vi "Kinetic Law Processor.vi"(5 "Kinetic Law":string, 11 "error in (no error)":errorcluster) -> (4 "No. of Operators":i32, 6 "No. of Operands":i32, 8 "Parsed array":string[](array[string]), 10 "Tagged String":string, 15 "error out":errorcluster)   [LabVIEW 2014]
doc: "This VI takes \"kinetic Law\" (enclosed in <apply>, </apply> tags) as input and parse it with unique tags. Currently, following five math functions are supported:\n+, - , /, *, pow\n\nDesigned by HB\nhaba@dtu.dk"
panel:
  out "result":i32
  out "flag":i32
  out "Temp_Strng":string
  out "App_Cnt":i32
  # "SOP3 pow SOP4 * SOP5 / kr_f kr_r EOP5 LacI EOP4 nc EOP3"
  # "pow ( (kr_f/kr_r)*LacI, nc)"
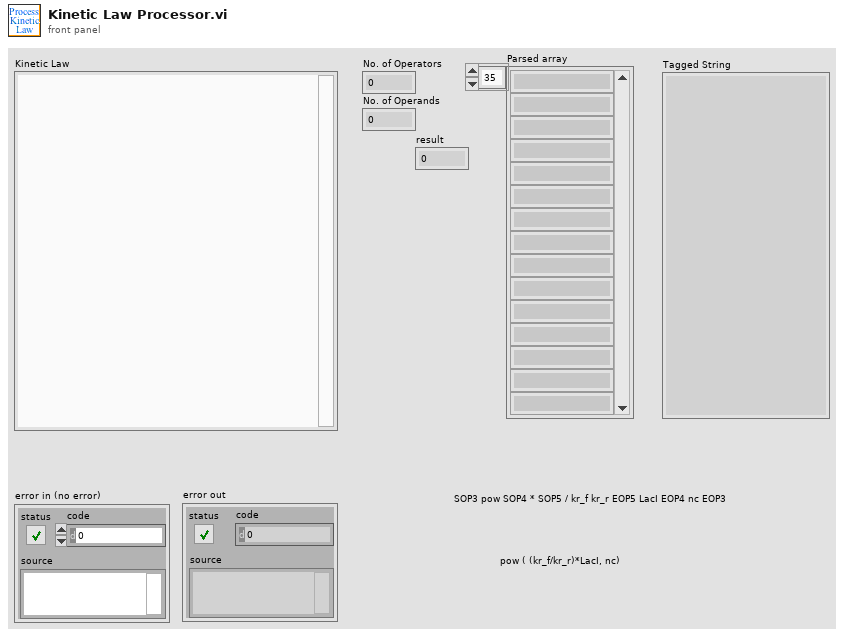
[diagram p1: front panel]
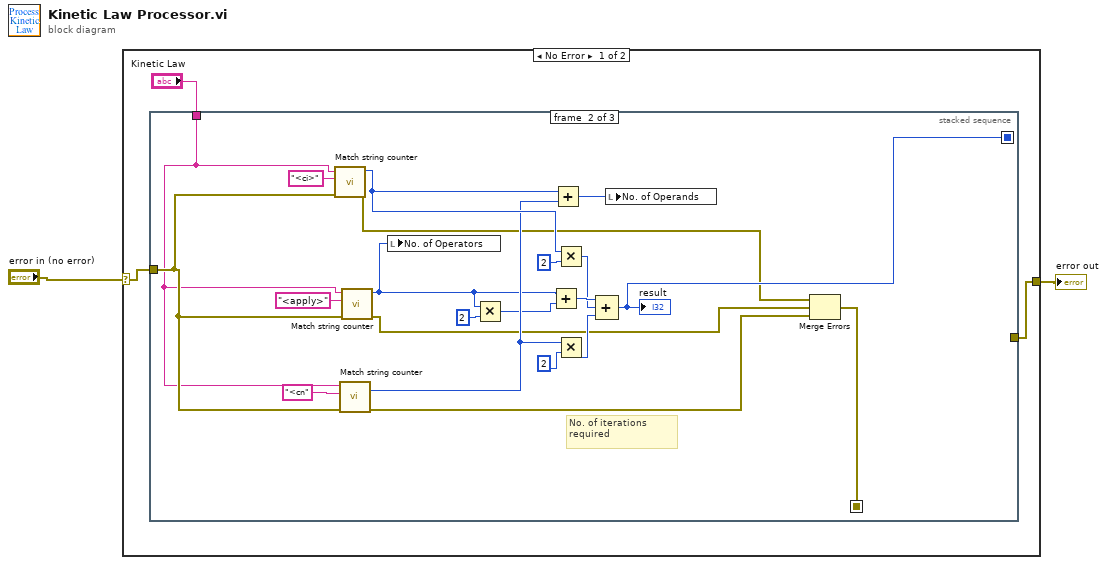
[diagram p0: block diagram]
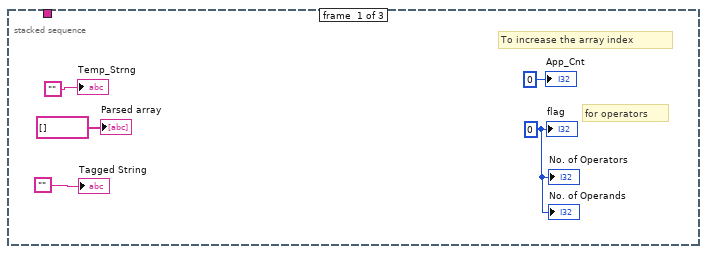
[diagram p2: hidden frame]
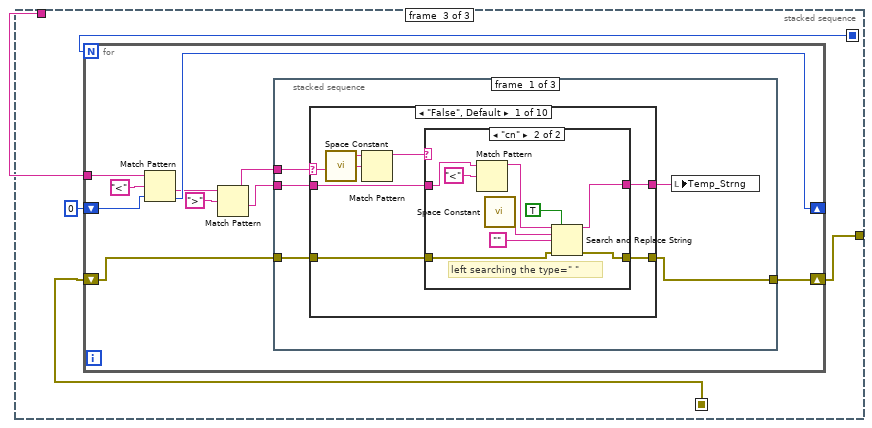
[diagram p3: hidden frame]
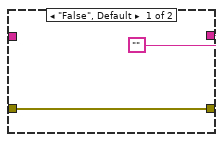
[diagram p4: hidden frame]
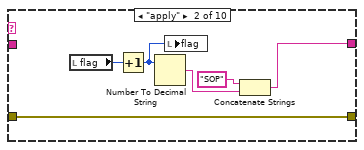
[diagram p5: hidden frame]
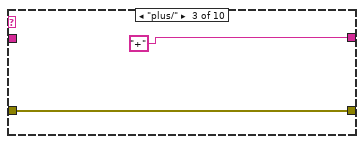
[diagram p6: hidden frame]
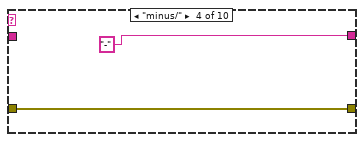
[diagram p7: hidden frame]
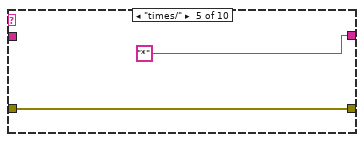
[diagram p8: hidden frame]
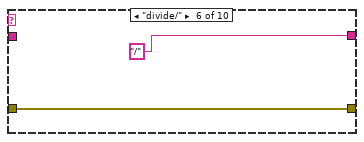
[diagram p9: hidden frame]
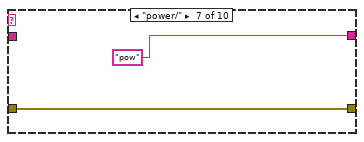
[diagram p10: hidden frame]
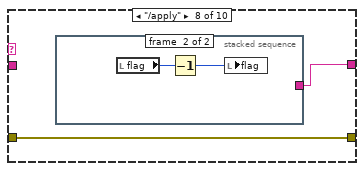
[diagram p11: hidden frame]
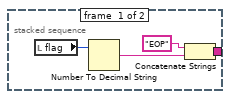
[diagram p12: hidden frame]
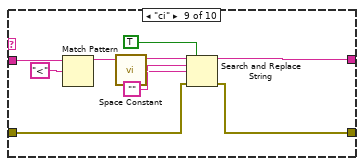
[diagram p13: hidden frame]
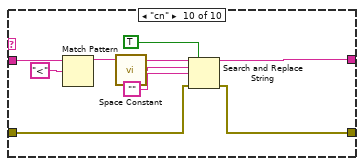
[diagram p14: hidden frame]
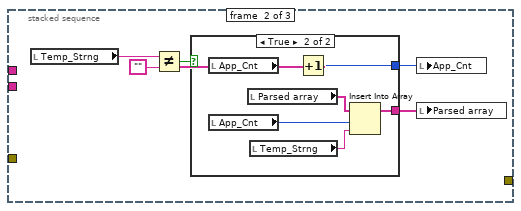
[diagram p15: hidden frame]
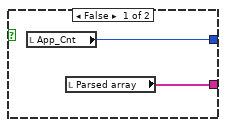
[diagram p16: hidden frame]
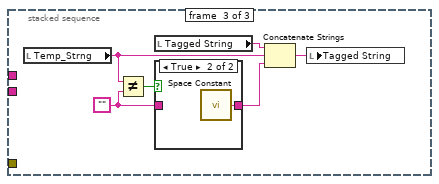
[diagram p17: hidden frame]
diagram:
  n1 = case shown="No Error" "error in (no error)" {
    selector: "error in (no error)" -> [w3 w133]
    tunnel: [w4 w133] -> w2
    frame No Error {
      n2 = stacked-sequence {
        seq-local: [_ w23 _] -> [_ _ w34]
        seq-local: [_ w12 _] -> [_ _ w33]
        tunnel: "Kinetic Law" -> [_ w11 w35]
        tunnel: w3 -> [_ w16 _]
        tunnel: [_ _ w32] -> w4
        frame #0 {
          w6 = 0 ("App_Cnt")
          # "To increase the array index"
          # "for operators"
          "App_Cnt" <- 0 ("App_Cnt")
          "Parsed array" <- string[] []
          "flag" <- w6
          "Temp_Strng" <- ""
          "Tagged String" <- ""
          "No. of Operators" <- w6
          "No. of Operands" <- w6
        }
        frame #1 {
          # "No. of iterations \nrequired"
          n3 = call "Match string counter.vi"("error in (no error)"=w16, "Match String"="<ci>", "Input string"=w11) -> ("error out"=w15:errorcluster, "Count"=w25:i32)  [unwired: 7 in]
          n4 = call "Match string counter.vi"("error in (no error)"=w16, "Match String"="<cn", "Input string"=w11) -> ("error out"=w13:errorcluster, "Count"=w24:i32)  [unwired: 7 in]
          n5 = call "Match string counter.vi"("error in (no error)"=w16, "Match String"="<apply>", "Input string"=w11) -> ("error out"=w14:errorcluster, "Count"=w17:i32)  [unwired: 7 in]
          n6 = local write "No. of Operators"(w17) -> ()
          n7 = Multiply(x=w17, y=2) -> (x*y=w18:i32)
          n8 = Add(x=w17, y=w18) -> (x+y=w30:i32)
          n9 = Add(x=w25, y=w24) -> (x+y=w22:i32)
          n10 = Multiply(x=w25, y=2) -> (x*y=w28:i32)
          n11 = Multiply(x=w24, y=2) -> (x*y=w26:i32)
          n12 = Compound Arithmetic op=ADD(w30, w28, w26) -> (w23:i32)
          "result" <- w23
          n13 = local write "No. of Operands"(w22) -> ()
          n14 = Merge Errors(w15, w14, w13) -> (w12:errorcluster)
        }
        frame #2 {
          n15 = for {
            N: w34 -> [_]
            tunnel: w35 -> [w45]
            shift-right: [w44] -> _
            shift-left: 0 ("offset past match") -> [w43]
            shift-right: [w37] -> w32
            shift-left: w33 -> [w38]
            n16 = Match Pattern(string=w45, regular expression="<" ("Match String"), offset (0)=w43) -> (after substring=w41:string, offset past match=w44:i32)  [unwired: 2 out]
            n17 = Match Pattern(string=w41, regular expression=">" ("Match String")) -> (before substring=w40:string, after substring=w39:string)  [unwired: 1 in, 2 out]
            n18 = stacked-sequence {
              tunnel: w40 -> [w51 _ _]
              tunnel: w39 -> [w50 _ _]
              tunnel: w38 -> [w48 _ _]
              tunnel: [w47 _ _] -> w37
              frame #0 {
                n19 = case shown="\"False\", Default" w51 {
                  selector: w51 -> [w56 _ _ _ _ _ _ _ _ _]
                  tunnel: [w58 w75 "+" "-" "*" "/" "pow" w87 w96 w105] -> w49
                  tunnel: w50 -> [w55 _ _ _ _ _ _ _ w101 w110]
                  tunnel: w48 -> [w53 w70 w76 w78 w80 w82 w84 w86 w95 w104]
                  tunnel: [w52 w70 w76 w78 w80 w82 w84 w86 w94 w103] -> w47
                  frame "False", Default {
                    n20 = call <vilib>:"Space Constant.vi"() -> ("String"=w57:string)
                    n21 = Match Pattern(string=w56, regular expression=w57) -> (before substring=w54:string)  [unwired: 1 in, 3 out]
                    n22 = case shown="\"cn\"" w54 {
                      tunnel: ["" w63] -> w58
                      tunnel: w55 -> [_ w64]
                      tunnel: w53 -> [w59 w62]
                      tunnel: [w59 w61] -> w52
                      frame "False", Default {
                      }
                      frame "cn" {
                        # "left searching the type=\" \""
                        n23 = Match Pattern(string=w64, regular expression="<" ("Match String")) -> (before substring=w69:string)  [unwired: 1 in, 3 out]
                        n24 = call <vilib>:"Space Constant.vi"() -> ("String"=w66:string)
                        n25 = Search and Replace String(replace all?=TRUE ("replace all? (F)"), input string=w69, search string=w66, replace string="" ("string"), error in=w62) -> (result string=w63:string, error out=w61:errorcluster)  [unwired: 3 in, 2 out]
                      }
                    }
                  }
                  frame "apply" {
                    n26 = local read "flag"() -> (w72:i32)
                    n27 = Increment(x=w72) -> (x+1=w73:i32)
                    n28 = Number To Decimal String(number=w73) -> (decimal integer string=w74:string)  [unwired: 1 in]
                    n29 = local write "flag"(w73) -> ()
                    n30 = Concatenate Strings("SOP", w74) -> (w75:string)
                  }
                  frame "plus/" {
                  }
                  frame "minus/" {
                  }
                  frame "times/" {
                  }
                  frame "divide/" {
                  }
                  frame "power/" {
                  }
                  frame "/apply" {
                    n31 = stacked-sequence {
                      tunnel: [w90 _] -> w87
                      frame #0 {
                        n32 = local read "flag"() -> (w88:i32)
                        n33 = Number To Decimal String(number=w88) -> (decimal integer string=w89:string)  [unwired: 1 in]
                        n34 = Concatenate Strings("EOP", w89) -> (w90:string)
                      }
                      frame #1 {
                        n35 = local read "flag"() -> (w92:i32)
                        n36 = Decrement(x=w92) -> (x-1=w93:i32)
                        n37 = local write "flag"(w93) -> ()
                      }
                    }
                  }
                  frame "ci" {
                    n38 = Match Pattern(string=w101, regular expression="<" ("Match String")) -> (before substring=w97:string)  [unwired: 1 in, 3 out]
                    n39 = call <vilib>:"Space Constant.vi"() -> ("String"=w100:string)
                    n40 = Search and Replace String(replace all?=TRUE ("replace all? (F)"), input string=w97, search string=w100, replace string="" ("string"), error in=w95) -> (result string=w96:string, error out=w94:errorcluster)  [unwired: 3 in, 2 out]
                  }
                  frame "cn" {
                    n41 = Match Pattern(string=w110, regular expression="<" ("Match String")) -> (before substring=w106:string)  [unwired: 1 in, 3 out]
                    n42 = call <vilib>:"Space Constant.vi"() -> ("String"=w109:string)
                    n43 = Search and Replace String(replace all?=TRUE ("replace all? (F)"), input string=w106, search string=w109, replace string="" ("string"), error in=w104) -> (result string=w105:string, error out=w103:errorcluster)  [unwired: 3 in, 2 out]
                  }
                }
                n44 = local write "Temp_Strng"(w49) -> ()
              }
              frame #1 {
                n45 = local read "Temp_Strng"() -> (w114:string)
                n46 = Not Equal?(x=w114, y="") -> (x != y?=w116:bool)
                n47 = case shown="True" w116 {
                  tunnel: [w117 w124] -> w113
                  tunnel: [w118 w123] -> w112
                  frame False {
                    n48 = local read "App_Cnt"() -> (w118:i32)
                    n49 = local read "Parsed array"() -> (w117:string[])
                  }
                  frame True {
                    n50 = local read "App_Cnt"() -> (w119:i32)
                    n51 = local read "App_Cnt"() -> (w121:i32)
                    n52 = local read "Parsed array"() -> (w122:string[])
                    n53 = local read "Temp_Strng"() -> (w120:string)
                    n54 = Increment(x=w119) -> (x+1=w123:i32)
                    n55 = Insert Into Array(array=w122, index=w121, new element=w120) -> (w124:string[])
                  }
                }
                n56 = local write "App_Cnt"(w112) -> ()
                n57 = local write "Parsed array"(w113) -> ()
              }
              frame #2 {
                w128 = ""
                n58 = local read "Temp_Strng"() -> (w125:string)
                n59 = Not Equal?(x=w125, y=w128) -> (x != y?=w129:bool)
                n60 = local read "Tagged String"() -> (w126:string)
                n61 = case shown="True" w129 {
                  tunnel: [w131 w132] -> w130
                  tunnel: w128 -> [w131 _]
                  frame False {
                  }
                  frame True {
                    n62 = call <vilib>:"Space Constant.vi"() -> ("String"=w132:string)
                  }
                }
                n63 = Concatenate Strings(w126, w125, w130) -> (w127:string)
                n64 = local write "Tagged String"(w127) -> ()
              }
            }
          }
        }
      }
    }
    frame Error {
    }
  }
  "error out" <- w2
